vi "Update Anlaysis Cluster error.vi"() -> (0 "error out":errorcluster, 4 "Path":path)   [LabVIEW 2020]
panel:
  out "appended array":string[][](array[string])
  in  "array":string[][](array[string])=[["Inst Array", "Port", "Inst type", "Units symbol", "Sampling Rate (Hz)", "Device ID", "Sync Delay (ms)", "Ch No", "Use latest Calib", "Calib filename", "Label", "X Pos", "Y Pos", "Z Pos", "Initial X", "Initial Y", "Initial Z", "Traverse Setup", "On Axes", "ADAM_Ch_Name", "Code name", "Metadata Ch Names", "Metadata Ch Values"], ["LDA", "", "LDA Vel", "U", "250.00", "LDA_IP.vi", "0.00", "0", "FALSE", "", "", "80.000", "0.000", "-105.002", "0.000", "0.000", "0.000", "Aero_Enclosure", "X Y Z", "", "1LDA:U", "", ""], ["LDA", "", "LDA Vel", "W", "250.00", "LDA_IP.vi", "0.00", "1", "FALSE", "", "", "0.000", "0.000", "0.000", "0.000", "0.000", "0.000", "Position N/A", "X Y Z", "", "2LDA:U", "", ""], ["Analogue", "COM18", "Raw with zero offsetting", "N01", "800.00", "Pressure_Multiplexer.vi", "0.00", "0", "FALSE", "", "N01", "0.000", "0.000", "1.000", "0.000", "0.000", "1.000", "No Traverse", "X Y Z", "", "1RZ:U", "", ""], ["Analogue", "COM18", "Raw with zero offsetting", "N02", "800.00", "Pressure_Multiplexer.vi", "0.00", "1", "FALSE", "", "N02", "0.004", "0.013", "1.000", "0.004", "0.013", "1.000", "No Traverse", "X Y Z", "", "2RZ:U", "", ""], ["Analogue", "COM18", "Raw with zero offsetting", "N04", "800.00", "Pressure_Multiplexer.vi", "0.00", "2", "FALSE", "", "N04", "0.015", "0.025", "1.000", "0.015", "0.025", "1.000", "No Traverse", "X Y Z", "", "3RZ:U", "", ""], ["Analogue", "COM18", "Raw with zero offsetting", "N06", "800.00", "Pressure_Multiplexer.vi", "0.00", "3", "FALSE", "", "N06", "0.032", "0.037", "1.000", "0.032", "0.037", "1.000", "No Traverse", "X Y Z", "", "4RZ:U", "", ""], ["Analogue", "COM18", "Raw with zero offsetting", "N07", "800.00", "Pressure_Multiplexer.vi", "0.00", "4", "FALSE", "", "N07", "0.057", "0.047", "1.000", "0.057", "0.047", "1.000", "No Traverse", "X Y Z", "", "5RZ:U", "", ""], ["Analogue", "COM18", "Raw with zero offsetting", "N09", "800.00", "Pressure_Multiplexer.vi", "0.00", "5", "FALSE", "", "N09", "0.089", "0.056", "1.000", "0.089", "0.056", "1.000", "No Traverse", "X Y Z", "", "6RZ:U", "", ""], ["Analogue", "COM18", "Raw with zero offsetting", "N10", "800.00", "Pressure_Multiplexer.vi", "0.00", "6", "FALSE", "", "N10", "0.126", "0.063", "1.000", "0.126", "0.063", "1.000", "No Traverse", "X Y Z", "", "7RZ:U", "", ""], ["Analogue", "COM18", "Raw with zero offsetting", "N11", "800.00", "Pressure_Multiplexer.vi", "0.00", "7", "FALSE", "", "N11", "0.168", "0.069", "1.000", "0.168", "0.069", "1.000", "No Traverse", "X Y Z", "", "8RZ:U", "", ""], ["Analogue", "COM18", "Raw with zero offsetting", "N13", "800.00", "Pressure_Multiplexer.vi", "0.00", "8", "FALSE", "", "N13", "0.216", "0.073", "1.000", "0.216", "0.073", "1.000", "No Traverse", "X Y Z", "", "9RZ:U", "", ""], ["Analogue", "COM18", "Raw with zero offsetting", "N14", "800.00", "Pressure_Multiplexer.vi", "0.00", "34", "FALSE", "", "N14", "0.268", "0.075", "1.000", "0.268", "0.075", "1.000", "No Traverse", "X Y Z", "", "10RZ:U", "", ""], ["Analogue", "COM18", "Raw with zero offsetting", "N15", "800.00", "Pressure_Multiplexer.vi", "0.00", "10", "FALSE", "", "N15", "0.323", "0.075", "1.000", "0.323", "0.075", "1.000", "No Traverse", "X Y Z", "", "11RZ:U", "", ""], ["Analogue", "COM18", "Raw with zero offsetting", "N16", "800.00", "Pressure_Multiplexer.vi", "0.00", "11", "FALSE", "", "N16", "0.380", "0.073", "1.000", "0.380", "0.073", "1.000", "No Traverse", "X Y Z", "", "12RZ:U", "", ""], ["Analogue", "COM18", "Raw with zero offsetting", "N18", "800.00", "Pressure_Multiplexer.vi", "0.00", "12", "FALSE", "", "N18", "0.440", "0.070", "1.000", "0.440", "0.070", "1.000", "No Traverse", "X Y Z", "", "13RZ:U", "", ""], ["Analogue", "COM18", "Raw with zero offsetting", "N19", "800.00", "Pressure_Multiplexer.vi", "0.00", "13", "FALSE", "", "N19", "0.500", "0.066", "1.000", "0.500", "0.066", "1.000", "No Traverse", "X Y Z", "", "14RZ:U", "", ""], ["Analogue", "COM18", "Raw with zero offsetting", "N20", "800.00", "Pressure_Multiplexer.vi", "0.00", "14", "FALSE", "", "N20", "0.587", "0.058", "1.000", "0.587", "0.058", "1.000", "No Traverse", "X Y Z", "", "15RZ:U", "", ""], ["Analogue", "COM18", "Raw with zero offsetting", "N22", "800.00", "Pressure_Multiplexer.vi", "0.00", "15", "FALSE", "", "N22", "0.671", "0.049", "1.000", "0.671", "0.049", "1.000", "No Traverse", "X Y Z", "", "16RZ:U", "", ""], ["Analogue", "COM18", "Raw with zero offsetting", "N23", "800.00", "Pressure_Multiplexer.vi", "0.00", "16", "FALSE", "", "N23", "0.750", "0.040", "1.000", "0.750", "0.040", "1.000", "No Traverse", "X Y Z", "", "17RZ:U", "", ""], ["Analogue", "COM18", "Raw with zero offsetting", "N24", "800.00", "Pressure_Multiplexer.vi", "0.00", "17", "FALSE", "", "N24", "0.821", "0.030", "1.000", "0.821", "0.030", "1.000", "No Traverse", "X Y Z", "", "18RZ:U", "", ""], ["Analogue", "COM18", "Raw with zero offsetting", "N26", "800.00", "Pressure_Multiplexer.vi", "0.00", "18", "FALSE", "", "N26", "0.883", "0.021", "1.000", "0.883", "0.021", "1.000", "No Traverse", "X Y Z", "", "19RZ:U", "", ""], ["Analogue", "COM18", "Raw with zero offsetting", "N27", "800.00", "Pressure_Multiplexer.vi", "0.00", "19", "FALSE", "", "N27", "0.933", "0.013", "1.000", "0.933", "0.013", "1.000", "No Traverse", "X Y Z", "", "20RZ:U", "", ""], ["Analogue", "COM18", "Raw with zero offsetting", "N29", "800.00", "Pressure_Multiplexer.vi", "0.00", "20", "FALSE", "", "N29", "0.970", "0.007", "1.000", "0.970", "0.007", "1.000", "No Traverse", "X Y Z", "", "21RZ:U", "", ""], ["Analogue", "COM18", "Raw with zero offsetting", "N30", "800.00", "Pressure_Multiplexer.vi", "0.00", "21", "FALSE", "", "N30", "1.000", "0.000", "1.000", "1.000", "0.000", "1.000", "No Traverse", "X Y Z", "", "22RZ:U", "", ""], ["Analogue", "COM18", "Raw with zero offsetting", "N28", "800.00", "Pressure_Multiplexer.vi", "0.00", "22", "FALSE", "", "N28", "0.953", "-0.010", "-1.000", "0.953", "-0.010", "-1.000", "No Traverse", "X Y Z", "", "23RZ:U", "", ""], ["Analogue", "COM18", "Raw with zero offsetting", "N25", "800.00", "Pressure_Multiplexer.vi", "0.00", "23", "FALSE", "", "N25", "0.821", "-0.030", "-1.000", "0.821", "-0.030", "-1.000", "No Traverse", "X Y Z", "", "24RZ:U", "", ""], ["Analogue", "COM18", "Raw with zero offsetting", "N21", "800.00", "Pressure_Multiplexer.vi", "0.00", "24", "FALSE", "", "N21", "0.629", "-0.054", "-1.000", "0.629", "-0.054", "-1.000", "No Traverse", "X Y Z", "", "25RZ:U", "", ""], ["Analogue", "COM18", "Raw with zero offsetting", "N17", "800.00", "Pressure_Multiplexer.vi", "0.00", "25", "FALSE", "", "N17", "0.413", "-0.072", "-1.000", "0.413", "-0.072", "-1.000", "No Traverse", "X Y Z", "", "26RZ:U", "", ""], ["Analogue", "COM18", "Raw with zero offsetting", "N12", "800.00", "Pressure_Multiplexer.vi", "0.00", "26", "FALSE", "", "N12", "0.213", "-0.073", "-1.000", "0.213", "-0.073", "-1.000", "No Traverse", "X Y Z", "", "27RZ:U", "", ""], ["Analogue", "COM18", "Raw with zero offsetting", "N08", "800.00", "Pressure_Multiplexer.vi", "0.00", "27", "FALSE", "", "N08", "0.067", "-0.050", "-1.000", "0.067", "-0.050", "-1.000", "No Traverse", "X Y Z", "", "28RZ:U", "", ""], ["Analogue", "COM18", "Raw with zero offsetting", "N05", "800.00", "Pressure_Multiplexer.vi", "0.00", "28", "FALSE", "", "N05", "0.021", "-0.030", "-1.000", "0.021", "-0.030", "-1.000", "No Traverse", "X Y Z", "", "29RZ:U", "", ""], ["Analogue", "COM18", "Raw with zero offsetting", "N03", "800.00", "Pressure_Multiplexer.vi", "0.00", "29", "FALSE", "", "N03", "0.004", "-0.014", "-1.000", "0.004", "-0.014", "-1.000", "No Traverse", "X Y Z", "", "30RZ:U", "", ""], ["Analogue", "COM23", "Generic Polynomial", "D", "5000.00", "Na-DAS_7609.vi", "0.00", "0", "FALSE", "Z:\\2021\\Aero_Tunnel\\Haydn Wootton\\Calibrations\\Cal_12-2021\\Laser Disp Volts to Angle2.xls", "", "0.000", "0.000", "0.000", "0.000", "0.000", "0.000", "Position N/A", "X Y Z", "", "1Gen:U", "", ""], ["Analogue", "COM23", "Raw voltage", "Sync", "5000.00", "Na-DAS_7609.vi", "0.00", "1", "FALSE", "", "", "0.000", "0.000", "0.000", "0.000", "0.000", "0.000", "Position N/A", "X Y Z", "", "1RV:U", "", ""]]
  out "Array":path[](array[path])
  out "File Changed":bool
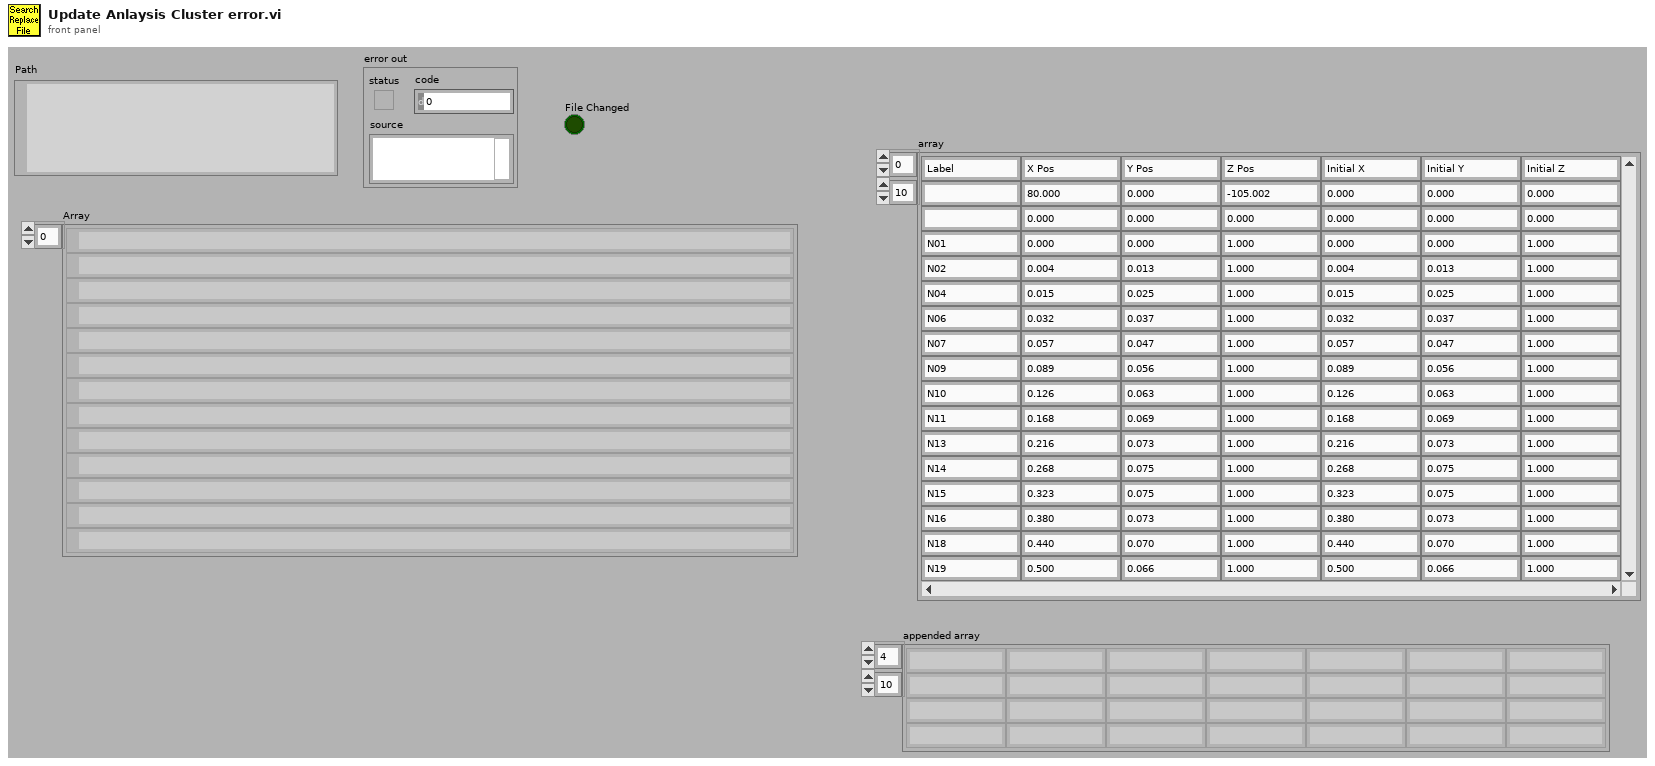
[diagram p1: front panel]
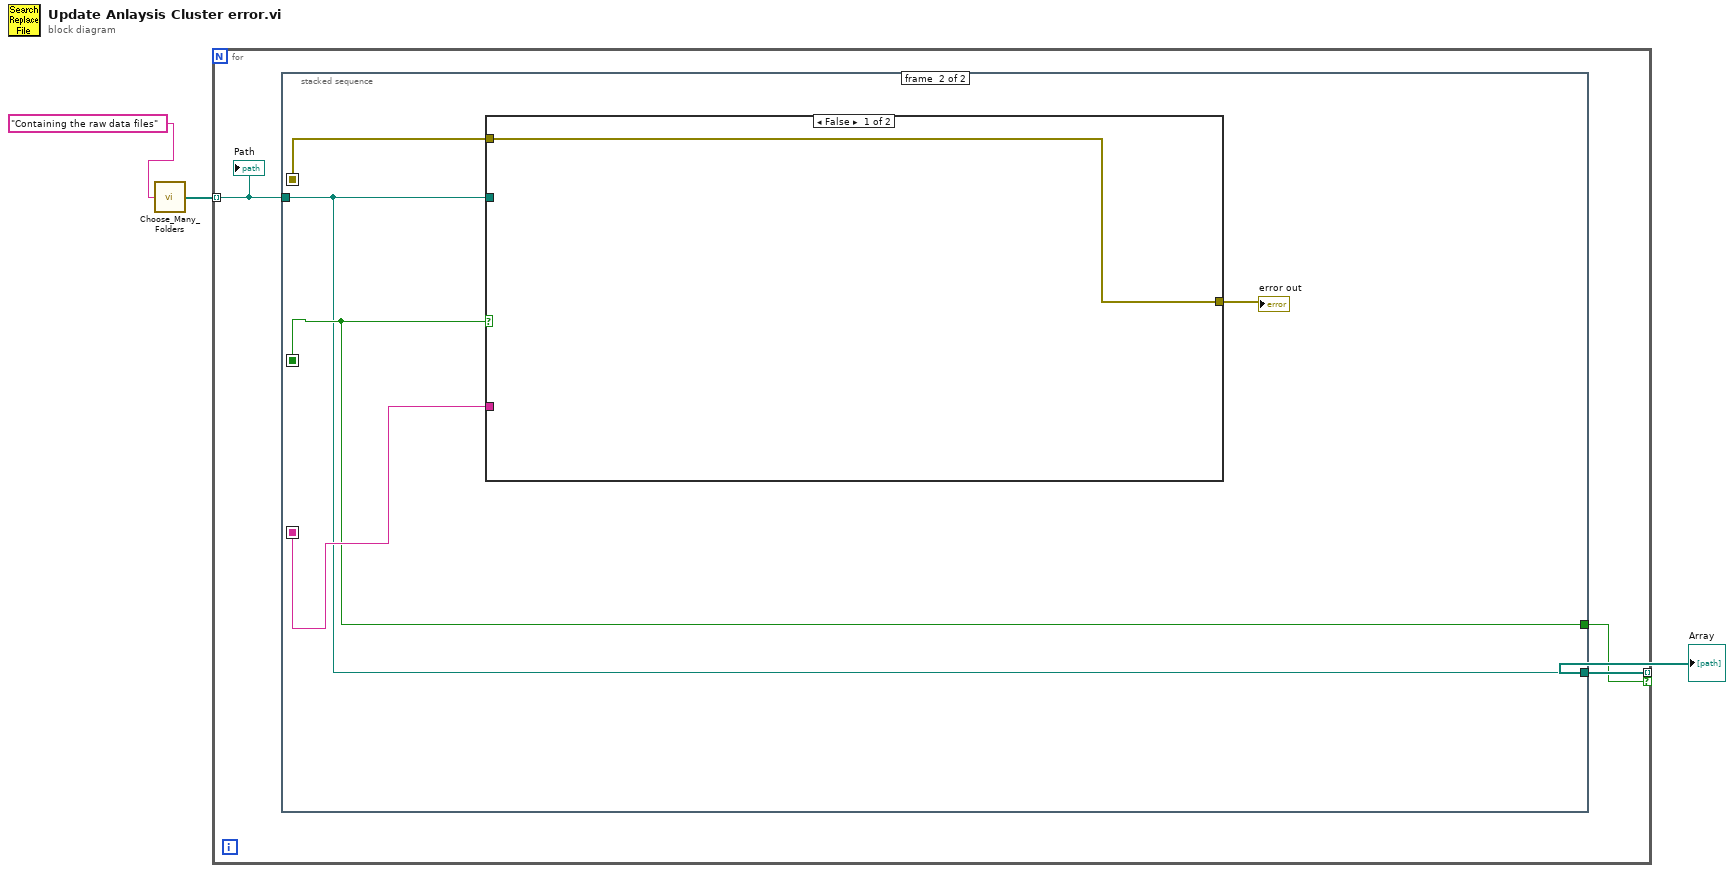
[diagram p0: block diagram]
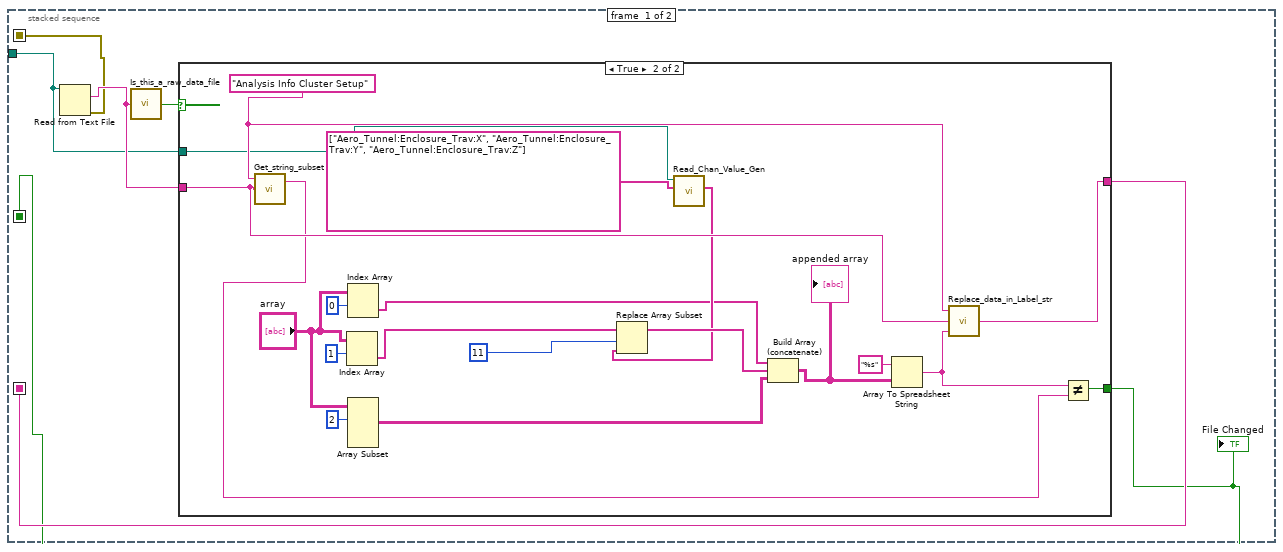
[diagram p2: hidden frame]
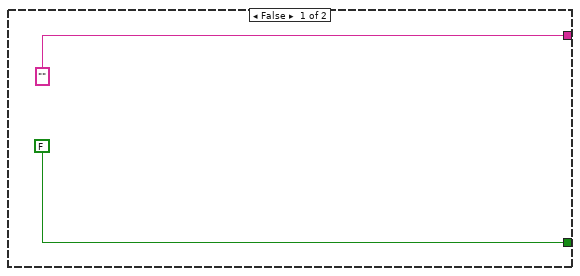
[diagram p3: hidden frame]
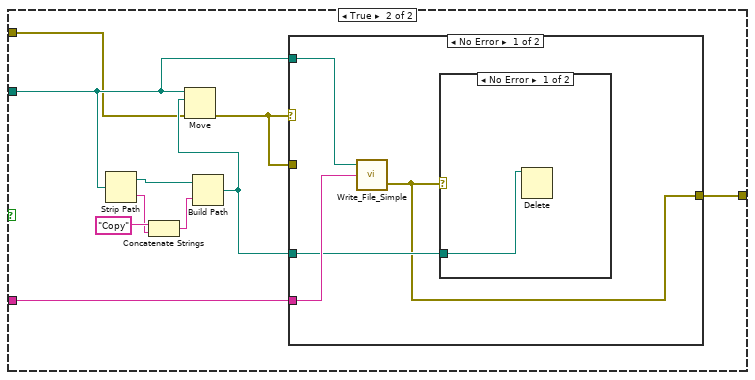
[diagram p4: hidden frame]
diagram:
  n1 = call "Choose_Many_Folders.vi"("Purpose of choosing folder"="Containing the raw data files") -> ("Files"=w2:path[])
  n2 = for {
    tunnel: w2 -> [w6] mode=indexing
    tunnel: [w5] -> w1 mode=indexing if=w4
    n3 = stacked-sequence {
      seq-local: [w8 _] -> [_ w38]
      seq-local: [w12 _] -> [_ w37]
      seq-local: [w11 _] -> [_ w36]
      tunnel: w6 -> [w7 w35]
      tunnel: [_ w35] -> w5
      tunnel: [_ w36] -> w4
      frame #0 {
        n4 = Read from Text File(file (use dialog)=w7) -> (text=w9:string, error out=w8:errorcluster)  [unwired: 3 in, 2 out]
        n5 = call "Is_this_a_raw_data_file.vi"("character string"=w9) -> ("Raw Dat File?"=w10:bool)  [unwired: 2 out]
        n6 = case shown="True" w10 {
          tunnel: ["" ("string") w31] -> w12
          tunnel: [FALSE w28] -> w11
          tunnel: w9 -> [_ w33]
          tunnel: w7 -> [_ w19]
          frame False {
          }
          frame True {
            w32 = "Analysis Info Cluster Setup"
            n7 = call "Get_string_subset.vi"("String to split"=w33, "File Label"=w32) -> ("Output string"=w29:string)  [unwired: 2 in, 1 out]
            n8 = Index Array(array="array", index (row)=1) -> (element=w25:string[])  [unwired: 1 in]
            n9 = Index Array(array="array", index (row)=0) -> (element=w15:string[])  [unwired: 1 in]
            n10 = Array Subset(array="array", index (row)=2 ("index")) -> (w22:string[][])  [unwired: 3 in]
            n11 = call "Read_Chan_Value_Gen.vi"("Desired Ch Names"=string[] ["Aero_Tunnel:Enclosure_Trav:X", "Aero_Tunnel:Enclosure_Trav:Y", "Aero_Tunnel:Enclosure_Trav:Z"], "Raw data file"=w19) -> ("Values"=w18:string[])  [unwired: 9 in]
            n12 = Replace Array Subset(array=w25, new element=w18, index=11) -> (w23:string[])
            n13 = Build Array (concatenate)(w15, w23, w22) -> (w21:string[][])
            "appended array" <- w21
            n14 = Array To Spreadsheet String(array=w21, 3:"%s" ("format string")) -> (spreadsheet string=w30:string)  [unwired: 1 in]
            n15 = call "Replace_data_in_Label_str.vi"("New data string"=w30, "Input string"=w33, "Variable name"=w32) -> ("Appended string"=w31:string)
            n16 = Not Equal?(x=w30, y=w29) -> (x != y?=w28:bool)
          }
        }
        "File Changed" <- w11
      }
      frame #1 {
        n17 = case shown="False" w36 {
          tunnel: w35 -> [_ w46]
          tunnel: w37 -> [_ w45]
          tunnel: [w40 w43] -> w39
          tunnel: w38 -> [w40 w41]
          frame False {
          }
          frame True {
            n18 = Strip Path(path=w46) -> (stripped path=w47:path, name=w49:string)
            n19 = Concatenate Strings("Copy" ("name or relative path"), w49) -> (w48:string)
            n20 = Build Path(base path=w47, name or relative path=w48) -> (appended path=w44:path)
            n21 = Move(source path=w46, error in=w41, 10:w44) -> (error out=w42:errorcluster)  [unwired: 2 in, 2 out]
            n22 = case shown="No Error" w42 {
              tunnel: w46 -> [w54 _]
              tunnel: w45 -> [w53 _]
              tunnel: w44 -> [w52 _]
              tunnel: [w51 w56] -> w43
              tunnel: w42 -> [_ w56]
              frame No Error {
                n23 = call "Write_File_Simple.vi"("character string"=w53, "file path"=w54) -> ("error out"=w51:errorcluster)  [unwired: 1 in, 1 out]
                n24 = case shown="No Error" w51 {
                  tunnel: w52 -> [w55 _]
                  frame No Error {
                    n25 = Delete(path (use dialog)=w55) -> ()  [unwired: 4 in, 3 out]
                  }
                  frame Error {
                  }
                }
              }
              frame Error {
              }
            }
          }
        }
        "error out" <- w39
      }
    }
    "Path" <- w6
  }
  "Array" <- w1
